vi "Create Config JSON.vi"() -> ()   [LabVIEW 2026]
uses:
  Plugin/AMS Climate Chamber Template/Configuration Params.ctl
  <vilib>/ADAS Replay HIL/Template Node/Plugin/Template Node/Common Configuration Params.ctl
  <vilib>/ADAS Replay HIL/AdasCommonUtilities/AdasCommonUtilities.lvlib
  8f15ed5a-ad49-4887-bb27-9da39d6e7646.vi
  C:/Program Files/National Instruments/AMS plugin/Capabilities/Capabilities/Utilities/Utilities.lvlib
  C:/Program Files/National Instruments/AMS plugin/Capabilities/Capabilities/High Level Capabilities/Climate Chamber Cluster/Climate Chamber Cluster.lvclass
  <vilib>/ADAS Replay HIL/Template Node/Plugin/Template Node/Template Node.lvclass
  Plugin/AMS Climate Chamber Template/AMS Climate Chamber Template.lvclass
panel:
  out "PAtools JSON":string
  in  "Create PAtools importable JSON?":bool=TRUE
  out "Version":string
  out "Generated JSON string":string
  out "error out":errorcluster
  in  "Custom Parameters":T1={"Common"={"Iteration Interval (s)"=0.01, "T0 (ns)"=0, "Priority"=100, "Processor"=-2, "Wait in Ready State"=TRUE}, "Amount of Channels"=1, "Address"="localhost"} {"Common"."Iteration Interval (s)" format="%#_13g"}
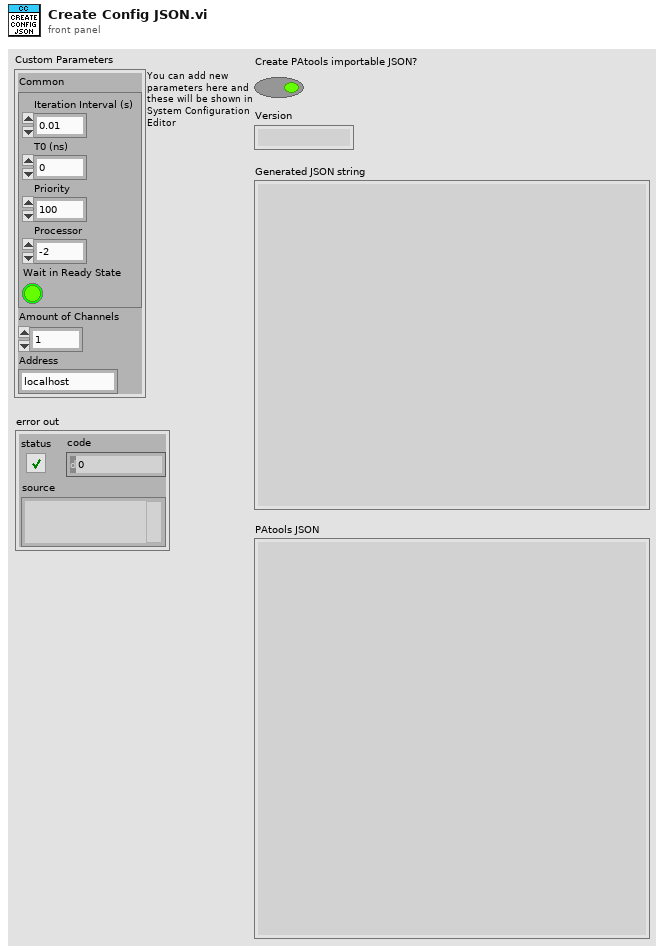
[diagram p1: front panel]
types:
  T1 = typedef "AMS Climate Chamber Template.lvlib/AMS Climate Chamber Template.lvclass/Configuration Params.ctl" = cluster{"Common":T2, "Amount of Channels":u32, "Address":string}
  T2 = typedef "Template Node.lvlib/Template Node.lvclass/Common Configuration Params.ctl" = cluster{"Iteration Interval (s)":dbl, "T0 (ns)":u64, "Priority":i32, "Processor":i32, "Wait in Ready State":bool}
  T3 = typedef "NI_App_Builder_API.lvlib/Build Specification Version.ctl" = cluster{"Major":u16, "Minor":u16, "Fix":u16, "Build":u16}
  T4 = typedef "Utilities.lvlib/Channel.ctl" = cluster{"Title":string, "SubTitle":string[], "Consumer?":bool, "Name":string, "Description":string, "Size":i32, "OffSets":i32[], "DataType":string[], "DefaultValue":dbl[]}
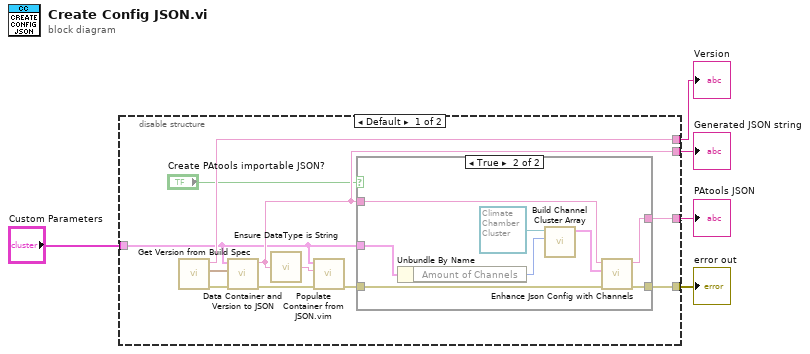
[diagram p0: block diagram]
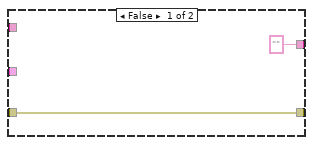
[diagram p2: hidden frame]
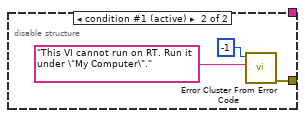
[diagram p3: hidden frame]
diagram:
  n1 = disable-structure shown="Default" {
    disable-tunnel: [w11 _] -> w5
    disable-tunnel: "Custom Parameters" -> [w9 _]
    disable-tunnel: [w7 w29] -> w3
    disable-tunnel: [w12 _] -> w2
    disable-tunnel: [w6 _] -> w1
    frame condition #0 {
      n2 = call "Get Version from Build Spec.vi"() -> ("error out"=w14:errorcluster, "Version"=w13:T3, "Version String"=w12:string)  [unwired: 8 in, 1 out]
      n3 = call <vilib>:"Data Container and Version to JSON.vi"("error in (no error)"=w14, "Version"=w13, "Container Variant"=w9) -> ("error out"=w16:errorcluster, "JSON string"=w11:string)  [unwired: 7 in]
      n4 = call <vilib>:"Ensure DataType is String.vi"("JSON In"=w11) -> ("JSON out"=w15:string)
      n5 = call "Populate Container from JSON.vim"("error in (no error)"=w16, "JSON string In"=w15, "Container In"=w9) -> ("error out"=w8:errorcluster)  [unwired: 6 in, 2 out]
      n6 = case shown="True" "Create PAtools importable JSON?" {
        tunnel: w11 -> [_ w26]
        tunnel: w9 -> [_ w25]
        tunnel: w8 -> [w18 w24]
        tunnel: [w18 w23] -> w7
        tunnel: ["" ("PAtools JSON") w22] -> w6
        frame False {
        }
        frame True {
          n7 = Unbundle By Name(w25) -> ("Amount of Channels"=w21:u32)
          n8 = call-dynamic "Build Channel Cluster Array.vi"("Climate Chamber Cluster.lvclass in"=refnum<class "Climate Chamber Cluster.lvclass"> refnum ("Climate Chamber Cluster.lvclass"), "Channels Amount"=w21) -> ("Channels out"=w20:cluster{"Channels":T4[]})  [unwired: 8 in]
          n9 = call "Enhance Json Config with Channels.vi"("error in"=w24, "Channels"=w20, "Json Config"=w26) -> ("error out"=w23:errorcluster, "PAtools JSON"=w22:string)  [unwired: 7 in]
        }
      }
    }
    frame condition #1 (active) {
      n10 = call <vilib>:"Error Cluster From Error Code.vi"("error message (\"\")"="This VI cannot run on RT. Run it under \"My Computer\"." ("error message (\"\")"), "error code (0)"=-1) -> ("error out"=w29:errorcluster)  [unwired: 7 in]
    }
  }
  "Generated JSON string" <- w5
  "error out" <- w3
  "Version" <- w2
  "PAtools JSON" <- w1
